vi "RT_Angle_Of_Attack_in_DLR_Navigation_Reference_System_v2(SubVI).vi"(6 "q":dbl[](array[numeric]), 8 "i":i32, 9 "V_wind [m/s]":dbl[][](array[numeric]), 10 "V (m/s)":dbl[](array[numeric])) -> (0 "Stream_direction [rad]":dbl[](array[numeric]), 2 "AoA_yaw (rad)":dbl, 3 "AoA_pitch (rad)":dbl)   [LabVIEW 2011]
uses:
  <vilib>/Analysis/_algsub.llb/Vector Norm Type.ctl
  <vilib>/Analysis/coordinate.llb/Euler Rotation Order.ctl
  <vilib>/Analysis/_algsub.llb/Real Vector Norm.vi
  <vilib>/Analysis/NI_AALPro.lvlib
panel:
  out "Elevation [deg]":dbl
  out "Azimuth [deg]":dbl
  out "AoA_yaw (deg)":dbl
  out "AoA_pitch (deg)":dbl
  out "appended array":dbl[](array[numeric])
  out "Speed_quat":dbl[](array[numeric])
  out "pitch_stream (rad)":dbl
  out "yaw_stream (rad)":dbl
  out "VV":dbl[](array[numeric])
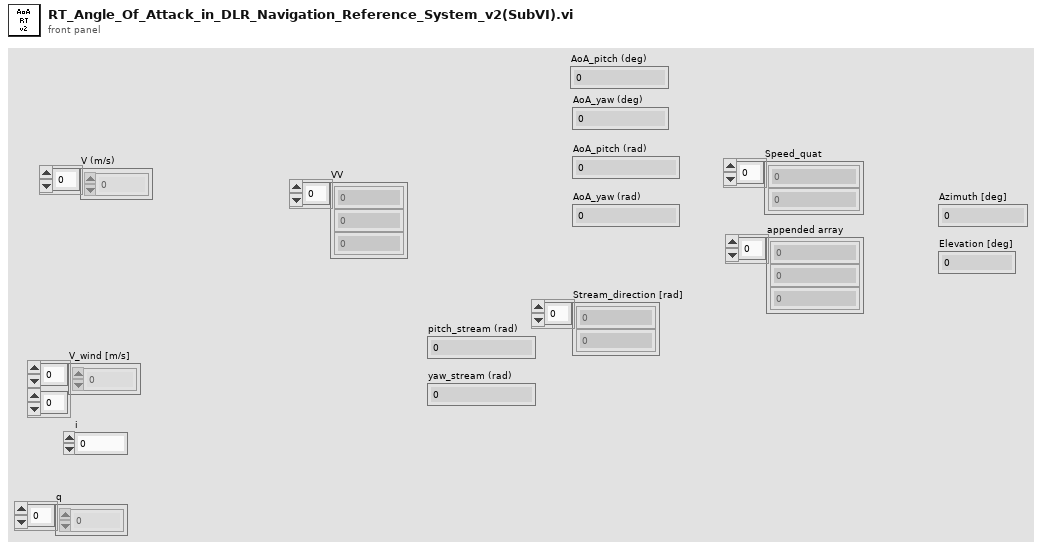
[diagram p1: front panel]
types:
  T1 = typedef "NI_AALPro.lvlib/Euler Rotation Order.ctl" = u16
  T2 = typedef "NI_AALPro.lvlib/Vector Norm Type.ctl" = u16
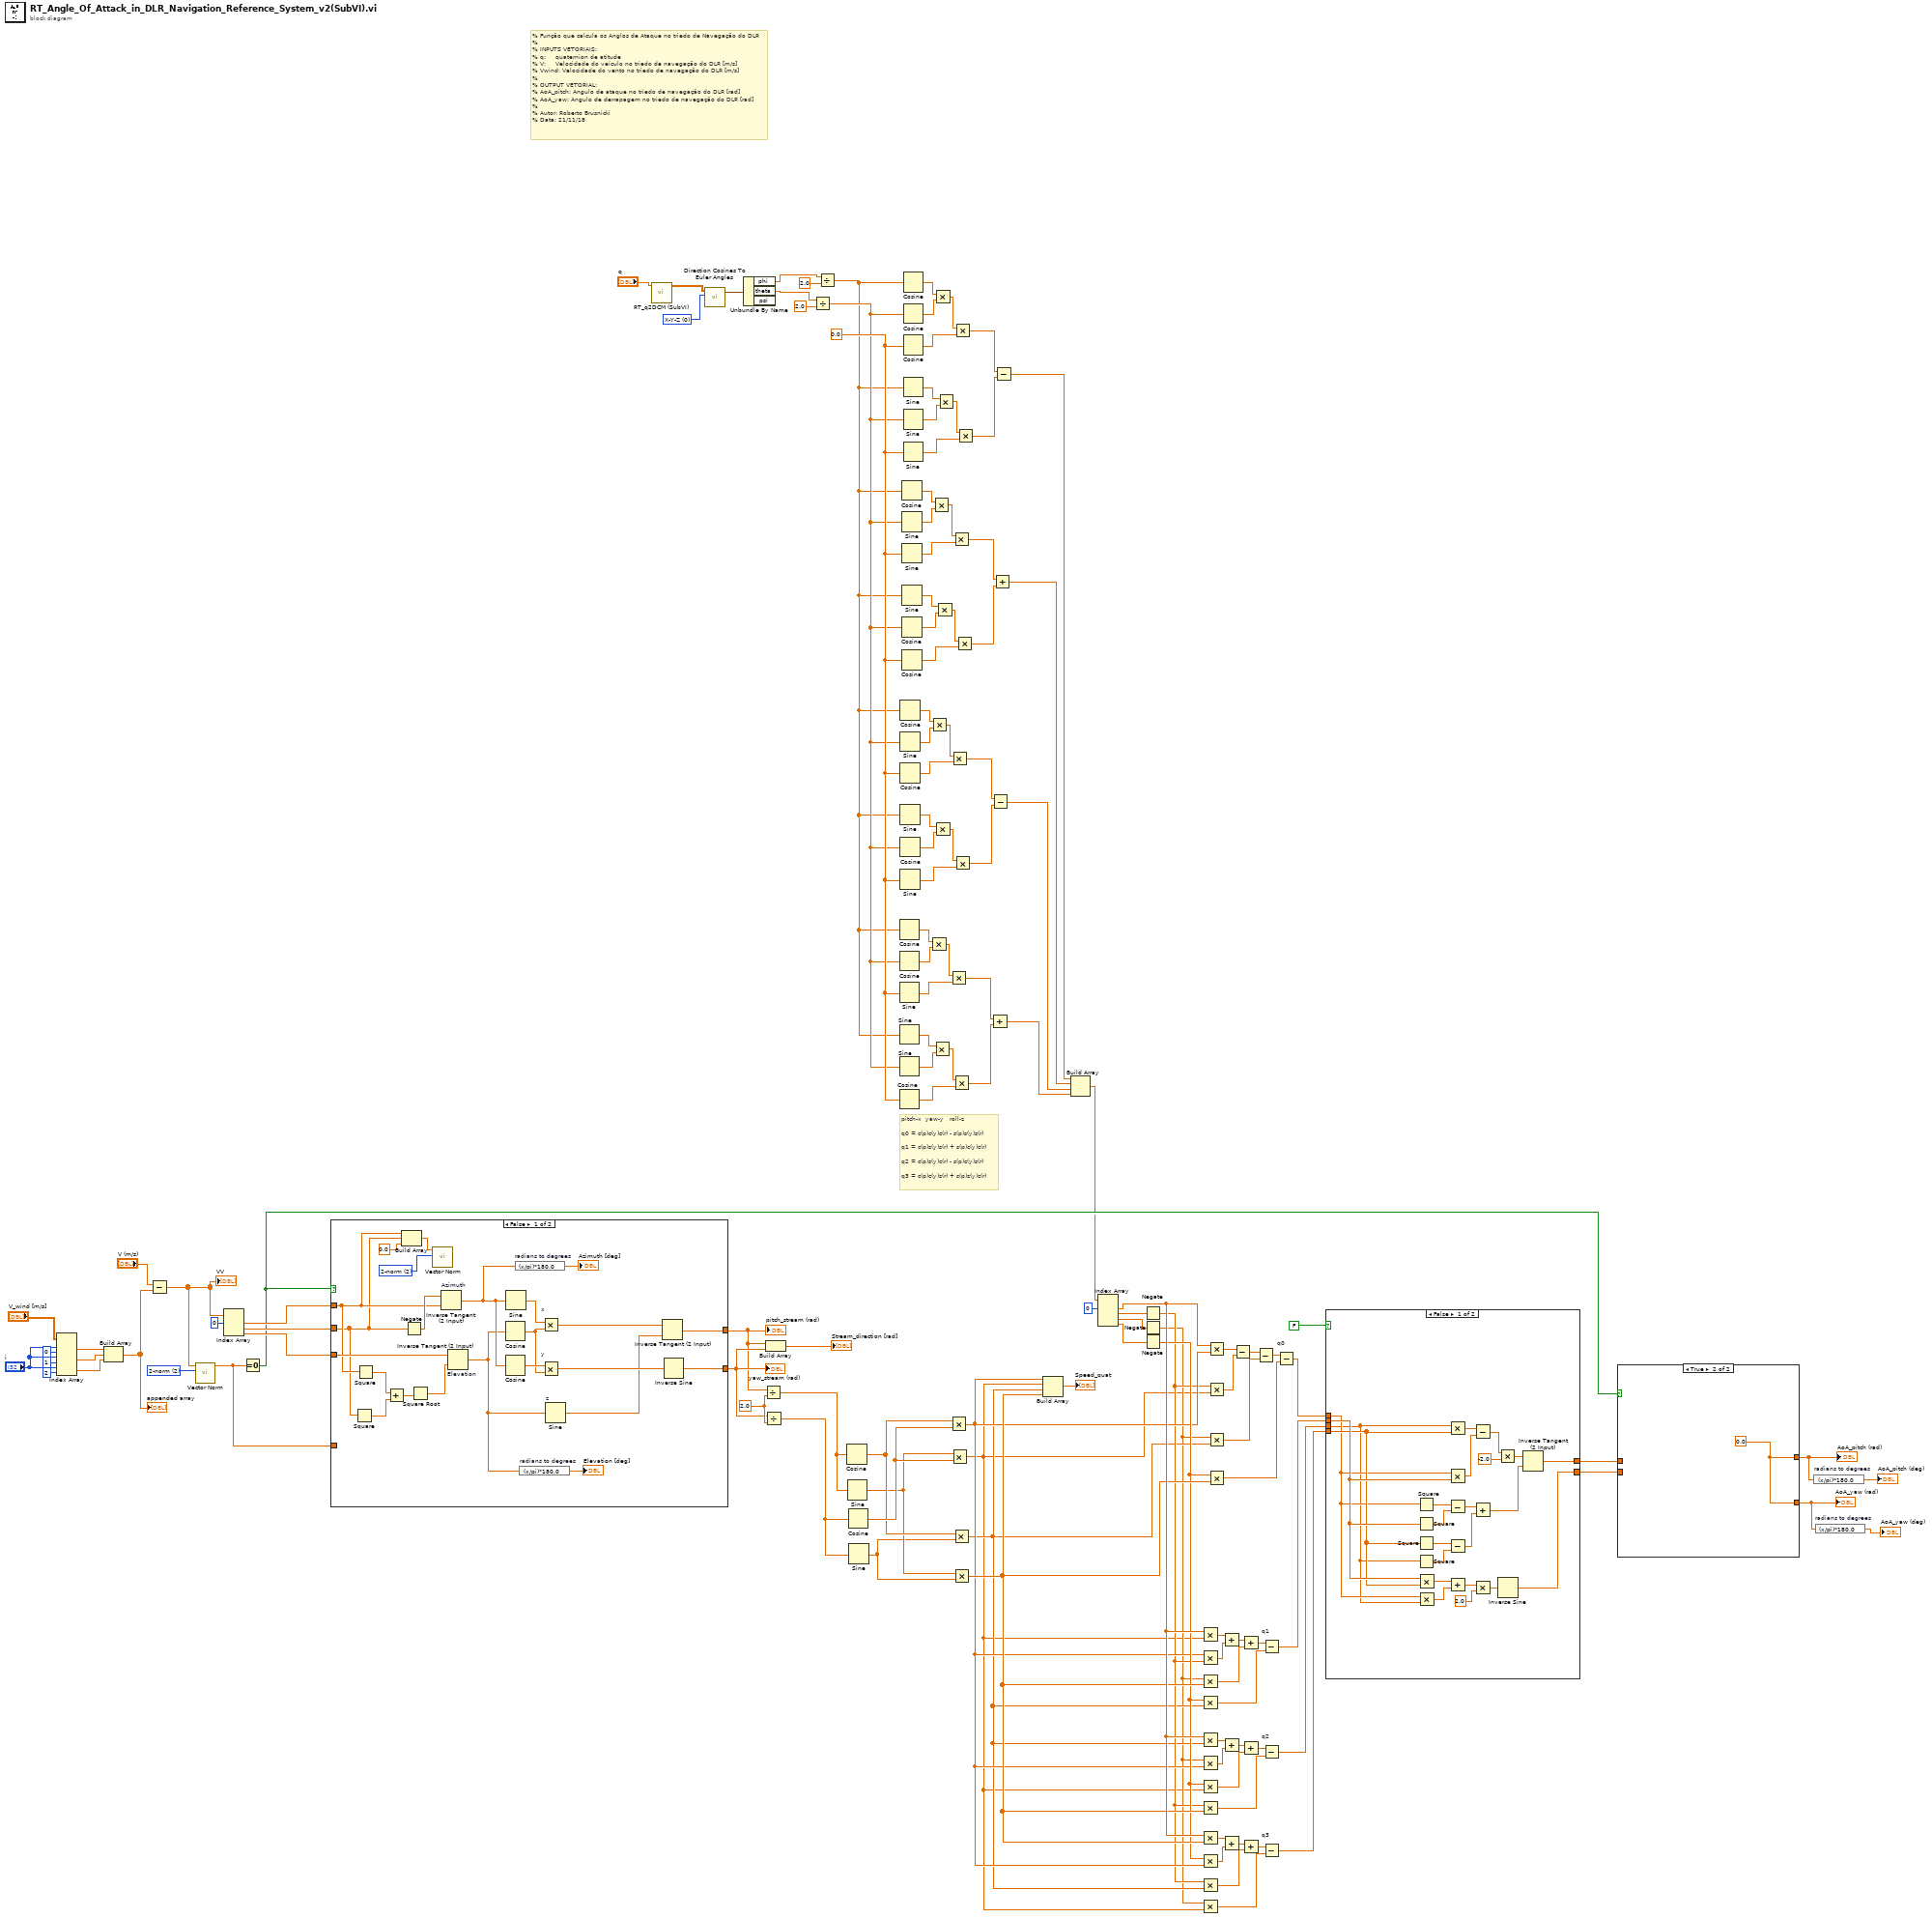
[diagram p0: block diagram]
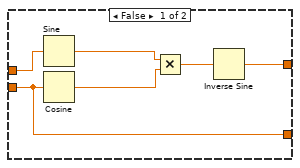
[diagram p2: hidden frame]
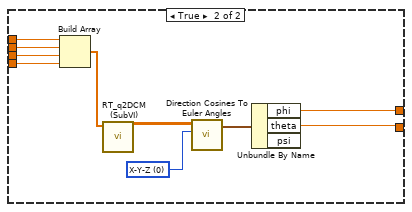
[diagram p3: hidden frame]
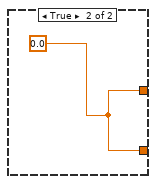
[diagram p4: hidden frame]
diagram:
  w14 = 0.0 ("x")
  w56 = T1 0 items=["X-Y-Z", "X-Z-Y", "Y-X-Z", "Y-Z-X", "Z-X-Y", "Z-Y-X", "X-Y-X", "X-Z-X", "Y-X-Y", "Y-Z-Y", "Z-X-Z", "Z-Y-Z"] ("rotation order")
  w116 = 2.0 ("y")
  w122 = T2 2 items=["1-norm"=1, "2-norm"=2, "Inf-norm"=3, "-Inf-norm"=4, "User Defined"=5] ("norm type")
  # "pitch-x  yaw-y   roll-z\n\nq0 = c(p)c(y)c(r) - s(p)s(y)s(r)\n\nq1 = c(p)s(y)s(r) + s(p)c(y)c(r)\n\nq2 = c(p)s(y)c(r) - s(p)c(y)s(r)\n\nq3 = c(p)c(y)s(r) + s(p)s(y)c(r)"
  # "% Função que calcula os Anglos de Ataque no triedo de Navegação do DLR \n%\n% INPUTS VETORIAIS: \n% q:     quaternion de atitude   \n% V:     Velocidade do veículo no triedo de navegação do DLR [m/s]\n% Vwind: Velocidade do vento no triedo de navegação do DLR [m/s]\n%\n% OUTPUT VETORIAL:\n% AoA_pitch: Angulo de ataque no triedo de navegação do DLR [rad]\n% AoA_yaw: Angulo de derrapagem no triedo de navegação do DLR [rad]\n%\n% Autor: Roberto Brusnicki\n% Data: 21/11/18"
  n1 = Index Array(array="V_wind [m/s]", index (row) #1="i", index (col) #1=0 ("disabled index (col)"), index (row) #2="i", index (col) #2=1 ("disabled index (col)"), index (row) #3="i", index (col) #3=2 ("disabled index (col)")) -> (element #1=w126:dbl, element #2=w125:dbl, element #3=w124:dbl)
  n2 = Build Array(w126, w125, w124) -> (w123:dbl[])
  "appended array" <- w123
  n3 = Subtract(x="V (m/s)", y=w123) -> (x-y=w121:dbl[])
  "VV" <- w121
  n4 = call-poly <vilib>:"Vector Norm.vi"("norm type"=w122, "Input Vector"=w121) -> ("norm"=w118:dbl)  [unwired: 8 in, 1 out]
  n5 = Index Array(array=w121, index #1=0 ("index (row)")) -> (element #1=w120:dbl, element #2=w119:dbl, element #3=w65:dbl)  [unwired: 2 in]
  n6 = Equal To 0?(x=w118) -> (x = 0?=w63:bool)
  n7 = case shown="False" w63 {
    tunnel: [w146 w156] -> w115
    tunnel: [w143 w156] -> w114
    tunnel: w120 -> [w136 _]
    tunnel: w119 -> [w135 _]
    tunnel: w118 -> [_ _]
    tunnel: w65 -> [w154 _]
    frame False {
      w153 = T2 2 items=["1-norm"=1, "2-norm"=2, "Inf-norm"=3, "-Inf-norm"=4, "User Defined"=5] ("norm type")
      n8 = Square(x=w135) -> (x^2=w138:dbl)
      n9 = Square(x=w136) -> (x^2=w137:dbl)
      n10 = Add(x=w137, y=w138) -> (x+y=w134:dbl)
      n11 = Build Array(w136, w135, 0.0 ("element")) -> (w151:dbl[])
      n12 = Negate(x=w135) -> (-x=w155:dbl)
      n13 = Square Root(x=w134) -> (sqrt(x)=w133:dbl)
      n14 = call-poly <vilib>:"Vector Norm.vi"("norm type"=w153, "Input Vector"=w151) -> ()  [unwired: 8 in, 2 out]
      n15 = Inverse Tangent (2 Input) "Azimuth"(1:w136, 2:w155) -> (0:w142:dbl)
      n16 = Inverse Tangent (2 Input) "Elevation"(1:w133, 2:w154) -> (0:w139:dbl)
      n17 = Cosine(x=w139) -> (cos(x)=w148:dbl)
      n18 = Cosine(x=w142) -> (cos(x)=w149:dbl)
      n19 = Sine(x=w142) -> (sin(x)=w150:dbl)
      n20 = expression code="(x/pi)*180.0" "radians to degrees"(w142) -> (→"Azimuth [deg]":dbl)
      n21 = expression code="(x/pi)*180.0" "radians to degrees"(w139) -> (→"Elevation [deg]":dbl)
      n22 = Multiply "x"(x=w150, y=w148) -> (x*y=w145:dbl)
      n23 = Multiply "y"(x=w149, y=w148) -> (x*y=w147:dbl)
      n24 = Sine "z"(x=w139) -> (sin(x)=w144:dbl)
      n25 = Inverse Tangent (2 Input)(1:w144, 2:w145) -> (0:w143:dbl)
      n26 = Inverse Sine(1:w147) -> (0:w146:dbl)
    }
    frame True {
      w156 = 0.0 ("Speed_pitch (rad)")
    }
  }
  "pitch_stream (rad)" <- w114
  "yaw_stream (rad)" <- w115
  n27 = call "RT_q2DCM (SubVI).vi"("Quaternion"="q") -> ("DCM"=w55:dbl[][])  [unwired: 10 in]
  n28 = call <vilib>:"Direction Cosines To Euler Angles.vi"("rotation order"=w56, "Direction Cosines"=w55) -> ("Euler Angles"=w57:cluster{"phi":dbl, "theta":dbl, "psi":dbl})  [unwired: 8 in, 1 out]
  n29 = Unbundle By Name(w57) -> ("phi"=w4:dbl, "theta"=w3:dbl)  [unwired: 1 out]
  n30 = Divide(x=w114, y=w116) -> (x/y=w113:dbl)
  n31 = Divide(x=w115, y=w116) -> (x/y=w112:dbl)
  n32 = Build Array(w114, w115) -> (→"Stream_direction [rad]":dbl[])
  n33 = Divide(x=w3, y=2.0) -> (x/y=w2:dbl)
  n34 = Divide(x=w4, y=2.0) -> (x/y=w1:dbl)
  n35 = Cosine(x=w113) -> (cos(x)=w110:dbl)
  n36 = Sine(x=w113) -> (sin(x)=w109:dbl)
  n37 = Cosine(x=w112) -> (cos(x)=w111:dbl)
  n38 = Sine(x=w112) -> (sin(x)=w108:dbl)
  n39 = Cosine(x=w1) -> (cos(x)=w15:dbl)
  n40 = Cosine(x=w2) -> (cos(x)=w16:dbl)
  n41 = Sine(x=w14) -> (sin(x)=w18:dbl)
  n42 = Sine(x=w1) -> (sin(x)=w20:dbl)
  n43 = Sine(x=w2) -> (sin(x)=w21:dbl)
  n44 = Cosine(x=w14) -> (cos(x)=w22:dbl)
  n45 = Cosine(x=w1) -> (cos(x)=w34:dbl)
  n46 = Sine(x=w2) -> (sin(x)=w33:dbl)
  n47 = Cosine(x=w14) -> (cos(x)=w31:dbl)
  n48 = Sine(x=w1) -> (sin(x)=w29:dbl)
  n49 = Cosine(x=w2) -> (cos(x)=w28:dbl)
  n50 = Sine(x=w14) -> (sin(x)=w27:dbl)
  n51 = Cosine(x=w1) -> (cos(x)=w35:dbl)
  n52 = Sine(x=w2) -> (sin(x)=w36:dbl)
  n53 = Sine(x=w14) -> (sin(x)=w38:dbl)
  n54 = Sine(x=w1) -> (sin(x)=w40:dbl)
  n55 = Cosine(x=w2) -> (cos(x)=w41:dbl)
  n56 = Cosine(x=w14) -> (cos(x)=w42:dbl)
  n57 = Cosine(x=w1) -> (cos(x)=w54:dbl)
  n58 = Cosine(x=w2) -> (cos(x)=w53:dbl)
  n59 = Cosine(x=w14) -> (cos(x)=w51:dbl)
  n60 = Sine(x=w1) -> (sin(x)=w49:dbl)
  n61 = Sine(x=w2) -> (sin(x)=w48:dbl)
  n62 = Sine(x=w14) -> (sin(x)=w47:dbl)
  n63 = Multiply(x=w15, y=w16) -> (x*y=w17:dbl)
  n64 = Multiply(x=w34, y=w33) -> (x*y=w32:dbl)
  n65 = Multiply(x=w35, y=w36) -> (x*y=w37:dbl)
  n66 = Multiply(x=w20, y=w21) -> (x*y=w19:dbl)
  n67 = Multiply(x=w54, y=w53) -> (x*y=w52:dbl)
  n68 = Multiply(x=w29, y=w28) -> (x*y=w30:dbl)
  n69 = Multiply(x=w40, y=w41) -> (x*y=w39:dbl)
  n70 = Multiply(x=w49, y=w48) -> (x*y=w50:dbl)
  n71 = Multiply(x=w17, y=w18) -> (x*y=w23:dbl)
  n72 = Multiply(x=w110, y=w111) -> (x*y=w76:dbl)
  n73 = Multiply(x=w32, y=w31) -> (x*y=w26:dbl)
  n74 = Multiply(x=w109, y=w111) -> (x*y=w72:dbl)
  n75 = Multiply(x=w37, y=w38) -> (x*y=w43:dbl)
  n76 = Multiply(x=w110, y=w108) -> (x*y=w74:dbl)
  n77 = Multiply(x=w19, y=w22) -> (x*y=w24:dbl)
  n78 = Multiply(x=w109, y=w108) -> (x*y=w78:dbl)
  n79 = Multiply(x=w52, y=w51) -> (x*y=w46:dbl)
  n80 = Multiply(x=w30, y=w27) -> (x*y=w25:dbl)
  n81 = Multiply(x=w39, y=w42) -> (x*y=w44:dbl)
  n82 = Multiply(x=w50, y=w47) -> (x*y=w45:dbl)
  n83 = Add(x=w23, y=w24) -> (x+y=w10:dbl)
  n84 = Subtract(x=w26, y=w25) -> (x-y=w11:dbl)
  n85 = Add(x=w43, y=w44) -> (x+y=w12:dbl)
  n86 = Subtract(x=w46, y=w45) -> (x-y=w13:dbl)
  n87 = Build Array(w76, w72, w74, w78) -> (→"Speed_quat":dbl[])
  n88 = Build Array(w13, w12, w11, w10) -> (w8:dbl[])
  n89 = Index Array(array=w8, index #1=0 ("index")) -> (element #1=w79:dbl, element #2=w104:dbl, element #3=w105:dbl, element #4=w106:dbl)  [unwired: 3 in]
  n90 = Negate(x=w104) -> (-x=w75:dbl)
  n91 = Negate(x=w105) -> (-x=w73:dbl)
  n92 = Negate(x=w106) -> (-x=w77:dbl)
  n93 = Multiply(x=w79, y=w72) -> (x*y=w97:dbl)
  n94 = Multiply(x=w76, y=w75) -> (x*y=w96:dbl)
  n95 = Multiply(x=w73, y=w78) -> (x*y=w93:dbl)
  n96 = Multiply(x=w77, y=w74) -> (x*y=w92:dbl)
  n97 = Multiply(x=w79, y=w74) -> (x*y=w86:dbl)
  n98 = Multiply(x=w73, y=w76) -> (x*y=w87:dbl)
  n99 = Multiply(x=w77, y=w72) -> (x*y=w90:dbl)
  n100 = Multiply(x=w75, y=w78) -> (x*y=w91:dbl)
  n101 = Multiply(x=w79, y=w78) -> (x*y=w85:dbl)
  n102 = Multiply(x=w77, y=w76) -> (x*y=w84:dbl)
  n103 = Multiply(x=w75, y=w74) -> (x*y=w81:dbl)
  n104 = Multiply(x=w73, y=w72) -> (x*y=w80:dbl)
  n105 = Multiply(x=w79, y=w76) -> (x*y=w103:dbl)
  n106 = Multiply(x=w75, y=w72) -> (x*y=w102:dbl)
  n107 = Multiply(x=w73, y=w74) -> (x*y=w100:dbl)
  n108 = Multiply(x=w77, y=w78) -> (x*y=w98:dbl)
  n109 = Add(x=w97, y=w96) -> (x+y=w95:dbl)
  n110 = Add(x=w86, y=w87) -> (x+y=w88:dbl)
  n111 = Add(x=w85, y=w84) -> (x+y=w83:dbl)
  n112 = Subtract(x=w103, y=w102) -> (x-y=w101:dbl)
  n113 = Add(x=w95, y=w93) -> (x+y=w94:dbl)
  n114 = Add(x=w88, y=w90) -> (x+y=w89:dbl)
  n115 = Add(x=w83, y=w81) -> (x+y=w82:dbl)
  n116 = Subtract(x=w101, y=w100) -> (x-y=w99:dbl)
  n117 = Subtract "q1"(x=w94, y=w92) -> (x-y=w70:dbl)
  n118 = Subtract "q2"(x=w89, y=w91) -> (x-y=w69:dbl)
  n119 = Subtract "q3"(x=w82, y=w80) -> (x-y=w68:dbl)
  n120 = Subtract "q0"(x=w99, y=w98) -> (x-y=w71:dbl)
  n121 = case shown="False" FALSE {
    tunnel: w71 -> [w164 w189]
    tunnel: w70 -> [w166 w188]
    tunnel: w69 -> [w163 w187]
    tunnel: w68 -> [w165 w186]
    tunnel: [w167 w184] -> w67
    tunnel: [w157 w183] -> w66
    frame False {
      n122 = Square(x=w164) -> (x^2=w174:dbl)
      n123 = Square(x=w166) -> (x^2=w173:dbl)
      n124 = Square(x=w165) -> (x^2=w172:dbl)
      n125 = Square(x=w163) -> (x^2=w171:dbl)
      n126 = Multiply(x=w166, y=w165) -> (x*y=w162:dbl)
      n127 = Multiply(x=w164, y=w163) -> (x*y=w161:dbl)
      n128 = Multiply(x=w163, y=w165) -> (x*y=w179:dbl)
      n129 = Multiply(x=w164, y=w166) -> (x*y=w178:dbl)
      n130 = Subtract(x=w174, y=w173) -> (x-y=w170:dbl)
      n131 = Subtract(x=w172, y=w171) -> (x-y=w169:dbl)
      n132 = Add(x=w162, y=w161) -> (x+y=w159:dbl)
      n133 = Subtract(x=w179, y=w178) -> (x-y=w177:dbl)
      n134 = Add(x=w170, y=w169) -> (x+y=w168:dbl)
      n135 = Multiply(x=w159, y=2.0) -> (x*y=w158:dbl)
      n136 = Multiply(x=w177, y=-2.0) -> (x*y=w175:dbl)
      n137 = Inverse Sine(1:w158) -> (0:w157:dbl)
      n138 = Inverse Tangent (2 Input)(1:w168, 2:w175) -> (0:w167:dbl)
    }
    frame True {
      w181 = T1 0 items=["X-Y-Z", "X-Z-Y", "Y-X-Z", "Y-Z-X", "Z-X-Y", "Z-Y-X", "X-Y-X", "X-Z-X", "Y-X-Y", "Y-Z-Y", "Z-X-Z", "Z-Y-Z"] ("rotation order")
      n139 = Build Array(w189, w188, w187, w186) -> (w185:dbl[])
      n140 = call "RT_q2DCM (SubVI).vi"("Quaternion"=w185) -> ("DCM"=w182:dbl[][])  [unwired: 10 in]
      n141 = call <vilib>:"Direction Cosines To Euler Angles.vi"("rotation order"=w181, "Direction Cosines"=w182) -> ("Euler Angles"=w180:cluster{"phi":dbl, "theta":dbl, "psi":dbl})  [unwired: 8 in, 1 out]
      n142 = Unbundle By Name(w180) -> ("phi"=w184:dbl, "theta"=w183:dbl)  [unwired: 1 out]
    }
  }
  n143 = case shown="True" w63 {
    tunnel: w67 -> [w195 _]
    tunnel: [w191 w196] -> w62
    tunnel: w66 -> [w190 _]
    tunnel: [w190 w196] -> w60
    frame False {
      n144 = Sine(x=w195) -> (sin(x)=w194:dbl)
      n145 = Cosine(x=w190) -> (cos(x)=w193:dbl)
      n146 = Multiply(x=w194, y=w193) -> (x*y=w192:dbl)
      n147 = Inverse Sine(1:w192) -> (0:w191:dbl)
    }
    frame True {
      w196 = 0.0
    }
  }
  "AoA_pitch (rad)" <- w62
  "AoA_yaw (rad)" <- w60
  n148 = expression code="(x/pi)*180.0" "radians to degrees"(w62) -> (→"AoA_pitch (deg)":dbl)
  n149 = expression code="(x/pi)*180.0" "radians to degrees"(w60) -> (→"AoA_yaw (deg)":dbl)
